vi "DoHandshake.vi"(4 "Error In":errorcluster, 5 "timeout ms (5000)":i32=5000, 7 "WebSocket Connection in":refnum<k5>) -> (0 "Error Out":errorcluster, 1 "Request URI":string, 2 "Header Array":cluster{"Name":string, "Value":string}[](array[cluster]), 3 "WebSocket Connection out":refnum<k5>)   [LabVIEW 2015, in "WebSockets.lvlib"]
doc: "Performs the WebSockets HTTP handshaking on the new TCP connection. The client sends HTTP headers and the server must reply with a correctly formed HTTP response.\nWebSockets API 1.3.0.13\nSam Sharp - Intelligent Energy\nCopyright (c) 2015, Intelligent Energy"
uses:
  WebSockets.lvlib
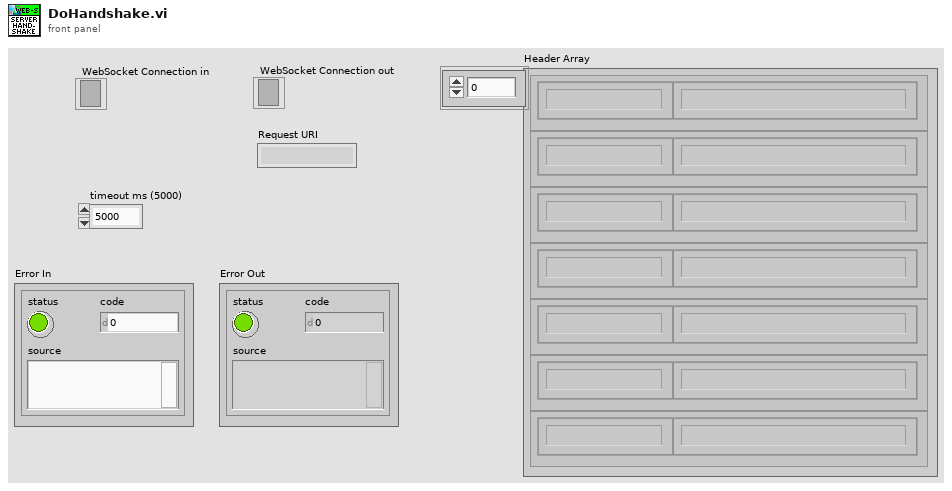
[diagram p1: front panel]
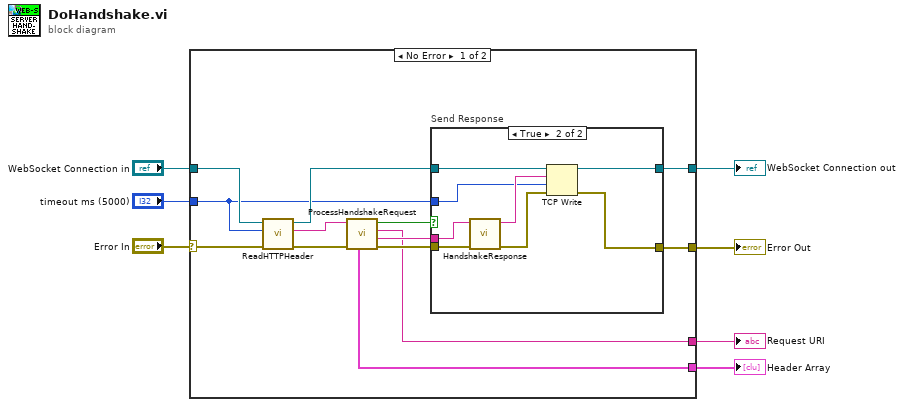
[diagram p0: block diagram]
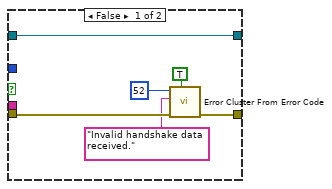
[diagram p2: hidden frame]
diagram:
  n1 = case shown="No Error" "Error In" {
    selector: "Error In" -> [w13 w36]
    tunnel: [w20 w35] -> w7
    tunnel: "WebSocket Connection in" -> [w14 w35]
    tunnel: [w16 w36] -> w4
    tunnel: "timeout ms (5000)" -> [w10 _]
    tunnel: [w8 _] -> w2
    tunnel: [w15 _] -> w1
    frame No Error {
      n2 = call "ReadHTTPHeader.vi"("error in (no error)"=w13, "timeout ms (25000)"=w10, "WebSocket Connection in"=w14) -> ("error out"=w12:errorcluster, "HTTP Header"=w9:string, "WebSocket Connection out"=w11:refnum<k5>)  [unwired: 2 in]
      n3 = call "ProcessHandshakeRequest.vi"("error in (no error)"=w12, "HTTP Headers"=w9) -> ("error out"=w17:errorcluster, "Sec-WebSocket-Key"=w19:string, "Path"=w15:string, "Is Websocket Request?"=w18:bool, "Header Array"=w8:cluster{"Name":string, "Value":string}[])  [unwired: 3 in, 2 out]
      n4 = case "Send Response" shown="True" w18 {
        tunnel: w19 -> [_ w34]
        tunnel: w11 -> [w26 w32]
        tunnel: [w26 w31] -> w20
        tunnel: w17 -> [w24 w29]
        tunnel: [w25 w28] -> w16
        tunnel: w10 -> [_ w27]
        frame False {
          n5 = call <vilib>:"Error Cluster From Error Code.vi"("show call chain? (False)"=TRUE, "error in (no error)"=w24, "error message (\"\")"="Invalid handshake data received." ("error message (\"\")"), "error code (0)"=52) -> ("error out"=w25:errorcluster)  [unwired: 5 in]
        }
        frame True {
          n6 = call "HandshakeResponse.vi"("error in (no error)"=w29, "Sec-WebSocket-Key"=w34) -> ("error out"=w30:errorcluster, "Response Headers"=w33:string)  [unwired: 4 in]
          n7 = TCP Write(connection ID=w32, data in=w33, error in (no error)=w30, 9:w27) -> (connection ID out=w31:refnum<k5>, error out=w28:errorcluster)  [unwired: 1 out]
        }
      }
    }
    frame Error {
    }
  }
  "WebSocket Connection out" <- w7
  "Error Out" <- w4
  "Header Array" <- w2
  "Request URI" <- w1
